vi "HTVacuum.constructor.vi"(0 "name":string, 2 "data in":string, 5 "error in (no error)":errorcluster) -> (14 "i ref out":refnum<vi>, 16 "data out":string, 19 "error out":errorcluster)   [LabVIEW 2014, in "HTVacuum.lvlib"]
doc: "This is the constructor of a class.\n\nLicense Agreement for this software:\n\nCopyright (C)\nGesellschaft für Schwerionenforschung, GSI\nPlanckstr. 1\n64291 Darmstadt\nGermany\n\nContact: D.Beck@gsi.de \n\nThis program is free software; you can redistribute it and/or modify it under the terms of the \nGNU General Public License as published by the Free Software Foundation; either version 2 of \nthe license, or (at your option) any later version.\n\nThis program is distributed in the hope that it will be useful, but WITHOUT ANY WARRANTY; \nwithout even the implied warranty of MERCHANTABILITY or FITNESS FOR A PARTICULAR PURPOSE. See the GNU General License for more details (http://www.gnu.org).\n\nGesellschaft für Schwerionenforschung, GSI\nPlanckstr. 1, 64291 Darmstadt, Germany\nFor all questions and ideas contact: M.Richter@gsi.de, H.Brand@gsi.de or D.Beck@gsi.de.\nLast update: 16-JUN-2004"
uses:
  HTVacuum.lvlib
  CSCore/CSApplicationBaseClasses/DeviceBase/DeviceBase.myEventNames.ctl
  CSinstr.lib/M&M/_ica01/ica-Lib SubVIs/M&M SubVIs/M&M USB init.vi
  CSCore/CSSystem/CSSystemLib/CSSystemLib.lvlib
  CSCore/BaseProcess/BaseProcess.lvlib
  CSCore/CSApplicationBaseClasses/DeviceBase/DeviceBase.lvlib
  CSCore/CSObj/CSObj.lvlib
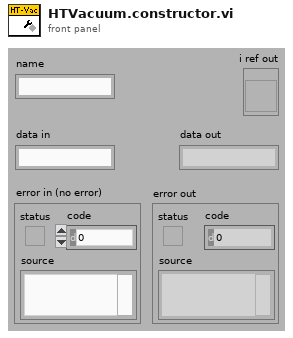
[diagram p1: front panel]
types:
  T1 = enum16{"SetAttribute", "GetAttribute", "CreateAttribute", "DestroyAttribute", "DestroyAllAtributes"}
  T2 = typedef "DeviceBase.lvlib/DeviceBase.myEventNames.ctl" = enum16{"lvmsg://Initialize", "lvmsg://Close", "lvmsg://Configure", "lvmsg://Reset", "lvmsg://IDQuery"}
  T3 = typedef "CSObj.lvlib/CSObj.i attribute.ctl" = cluster{"VI Refnum":refnum<vi>, "Front Panel Ref":refnum<vi>, "semaphore":T4, "date of birth":dbl, "ageID":i32, "systemID":i32, "classID":i32, "conditionID":i32, "DefaultPanelType":u16}
  T4 = typedef "Semaphore RefNum" = refnum<k1>
  T5 = typedef "BaseProcess.lvlib/BaseProcess.i attribute.ctl" = cluster{"EventStatus":string, "EventError":i32, "PresetEvtWatchD":i32, "PresetPdcWatchD":i32, "EventTimeout":i32, "PeriodicInterval":i32, "Interface":string[], "Address":string[], "Special":string[], "PeriodicError":i32, "PeriodicStatus":string, "SuperProc":string, "Descriptors":T6[], "CaseRef":refnum<vi>, "PdcRef":refnum<vi>, "Thread Ref":refnum<vi>, "eventErrorID":i32, "eventStatusID":i32, "periodicErrorID":i32, "periodicStatusID":i32, "pdcCtrID":i32}
  T6 = typedef "BaseProcess.lvlib/BaseProcess.descriptor definition.ctl" = cluster{"selector":string, "descriptor":T7}
  T7 = typedef "BaseProcess.lvlib/BaseProcess.descriptor string definition.ctl" = string
  T8 = typedef "HTVacuum.lvlib/HTVacuum.i attribute.ctl" = cluster{"USB-Handle":cluster{"Write handle":i32, "Read handle":i32}}
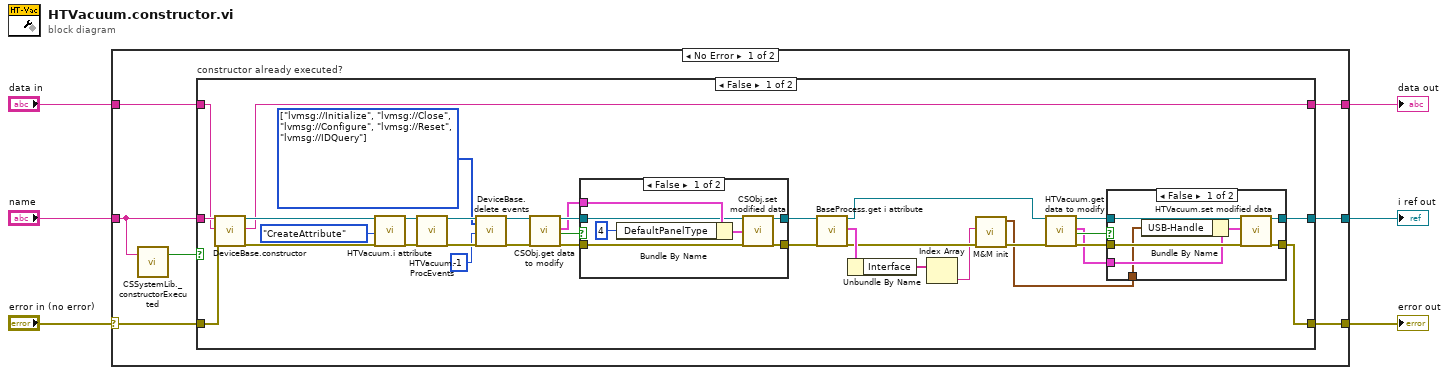
[diagram p0: block diagram]
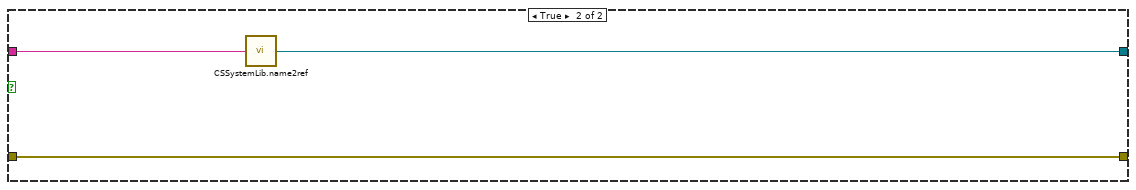
[diagram p4: hidden frame]
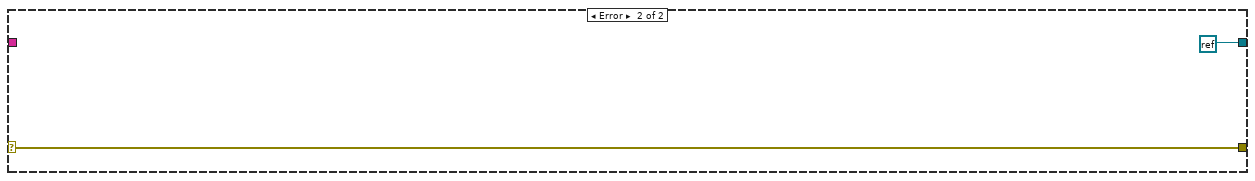
[diagram p5: hidden frame]
diagram:
  n1 = case shown="No Error" "error in (no error)" {
    selector: "error in (no error)" -> [w11 w69]
    tunnel: "name" -> [w10 _]
    tunnel: [w13 refnum<k0> refnum] -> w5
    tunnel: [w12 w69] -> w4
    tunnel: "data in" -> [w8 _]
    tunnel: [w7 _] -> w1
    frame No Error {
      n2 = call "CSSystemLib._constructorExecuted.vi"("name"=w10) -> ("constructor executed?"=w9:bool)  [unwired: 18 in]
      n3 = case "constructor already executed?" shown="False" w9 {
        tunnel: [w36 w67] -> w13
        tunnel: [w37 w66] -> w12
        tunnel: w11 -> [w30 w66]
        tunnel: w10 -> [w31 w68]
        tunnel: w8 -> [w29 _]
        tunnel: [w27 _] -> w7
        frame False {
          w22 = T2[] [enum."lvmsg://Initialize", enum."lvmsg://Close", enum."lvmsg://Configure", enum."lvmsg://Reset", enum."lvmsg://IDQuery"] items=["lvmsg://Initialize", "lvmsg://Close", "lvmsg://Configure", "lvmsg://Reset", "lvmsg://IDQuery"] ("events")
          n4 = call "DeviceBase.constructor.vi"("name"=w31, "data in"=w29, "error in (no error)"=w30) -> ("i ref out"=w28:refnum<vi>, "data out"=w27:string, "error out"=w26:errorcluster)  [unwired: 14 in]
          n5 = call "HTVacuum.i attribute.vi"("VI Refnum"=w28, "Action"=T1."CreateAttribute", "error in (no error)"=w26) -> ("VI Refnum out"=w46:refnum<vi>, "error out"=w45:errorcluster)  [unwired: 14 in, 1 out]
          n6 = call "HTVacuum.ProcEvents.vi"("i ref in"=w46, "error in (no error)"=w45) -> ("i ref out"=w24:refnum<vi>, "error out"=w25:errorcluster)  [unwired: 16 in]
          n7 = call "DeviceBase.delete events.vi"("i ref in"=w24, "events"=w22, "ms timeout (10000)"=-1, "error in (no error)"=w25) -> ("i ref out"=w18:refnum<vi>, "error out"=w17:errorcluster)  [unwired: 13 in, 1 out]
          n8 = call "CSObj.get data to modify.vi"("i ref in"=w18, "error in (no error)"=w17) -> ("i ref out"=w21:refnum<vi>, "i attribute"=w19:T3, "timed out"=w14:bool, "error out"=w20:errorcluster)  [unwired: 14 in]
          n9 = case shown="False" w14 {
            tunnel: [w52 w56] -> w16
            tunnel: w21 -> [w53 w56]
            tunnel: [w50 w55] -> w15
            tunnel: w20 -> [w51 w55]
            tunnel: w19 -> [w54 _]
            frame False {
              n10 = Bundle By Name(cluster=w54, "DefaultPanelType"=u16 4) -> (w49:T3)
              n11 = call "CSObj.set modified data.vi"("i ref in"=w53, "i attribute"=w49, "error in (no error)"=w51) -> ("i ref out"=w52:refnum<vi>, "error out"=w50:errorcluster)  [unwired: 15 in]
            }
            frame True {
            }
          }
          n12 = call "BaseProcess.get i attribute.vi"("i ref in"=w16, "error in (no error)"=w15) -> ("i ref out"=w39:refnum<vi>, "i attribute"=w43:T5, "error out"=w42:errorcluster)  [unwired: 15 in]
          n13 = Unbundle By Name(w43) -> ("Interface"=w44:string[])
          n14 = Index Array(array=w44) -> (element=w41:string)  [unwired: 1 in]
          n15 = call-poly "M&M init.vi"("error in (no error)"=w42, "Moritz-Serial# (no ID)"=w41) -> ("error out"=w40:errorcluster, "USB-Handles out"=w32:cluster{"Write handle":i32, "Read handle":i32})  [unwired: 6 in, 2 out]
          n16 = call "HTVacuum.get data to modify.vi"("i ref in"=w39, "error in (no error)"=w40) -> ("i ref out"=w35:refnum<vi>, "i attribute"=w33:T8, "timed out"=w34:bool, "error out"=w38:errorcluster)  [unwired: 14 in]
          n17 = case shown="False" w34 {
            tunnel: w38 -> [w63 w64]
            tunnel: [w62 w64] -> w37
            tunnel: [w61 w65] -> w36
            tunnel: w35 -> [w60 w65]
            tunnel: w33 -> [w59 _]
            tunnel: w32 -> [w57 _]
            frame False {
              n18 = Bundle By Name(cluster=w59, "USB-Handle"=w57) -> (w58:T8)
              n19 = call "HTVacuum.set modified data.vi"("i ref in"=w60, "i attribute"=w58, "error in (no error)"=w63) -> ("i ref out"=w61:refnum<vi>, "error out"=w62:errorcluster)  [unwired: 15 in]
            }
            frame True {
            }
          }
        }
        frame True {
          n20 = call "CSSystemLib.name2ref.vi"("name"=w68) -> ("obj refnum"=w67:refnum<vi>)
        }
      }
    }
    frame Error {
    }
  }
  "i ref out" <- w5
  "error out" <- w4
  "data out" <- w1
